vi "CAN Init.vi"(9 "pCanConfig":T1, 10 "CANIndex":u8, 11 "DevIndex":i32) -> (3 "function return":i32)   [LabVIEW 2010, in "usb2can.lvlib"]
doc: "int WINAPI CAN_Init(int DevIndex, unsigned char CANIndex, PCAN_INIT_CONFIG pCanConfig);"
uses:
  usb2can.lvlib
  USB2XXX.dll
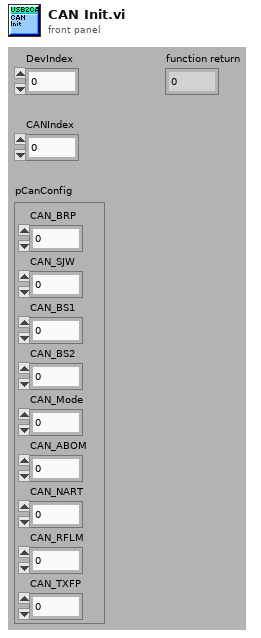
[diagram p1: front panel]
types:
  T1 = cluster{"CAN_BRP":u32, "CAN_SJW":u8, "CAN_BS1":u8, "CAN_BS2":u8, "CAN_Mode":u8, "CAN_ABOM":u8, "CAN_NART":u8, "CAN_RFLM":u8, "CAN_TXFP":u8}
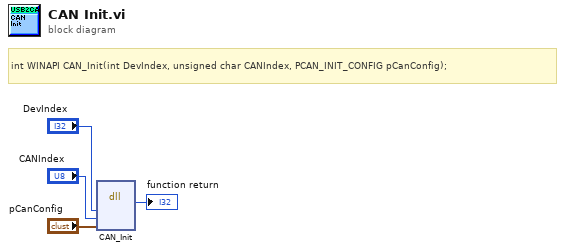
[diagram p0: block diagram]
diagram:
  # "int WINAPI CAN_Init(int DevIndex, unsigned char CANIndex, PCAN_INIT_CONFIG pCanConfig);"
  n1 = dll-call lib="G:/OtherWork/USB2XXX_Example/trunk/Labview/PublicFiles/usb2can/USB2XXX.*" fn="CAN_Init"("DevIndex"="DevIndex", "CANIndex"="CANIndex", "pCanConfig"="pCanConfig") -> (→"function return":i32)  [unwired: 6 in, 2 out]
